vi "getAll.vi"(8 "error in (no error)":errorcluster, 11 "Instrument.Oxford1820 in":refnum<class "Instrument.OxfordVRM.lvclass">) -> (0 "error out":errorcluster, 2 "getAll":variant, 3 "Instrument.Oxford1820 out":refnum<class "Instrument.OxfordVRM.lvclass">)   [LabVIEW 2016, in "Instrument.OxfordVRM.lvclass"]
uses:
  Instrument.OxfordVRM.lvclass
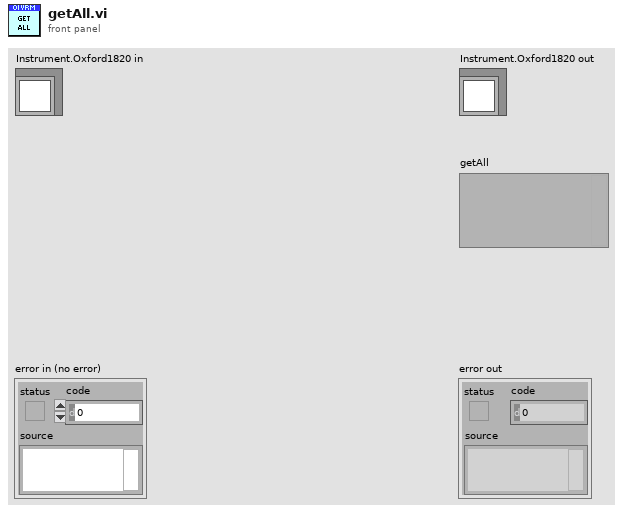
[diagram p1: front panel]
types:
  T1 = typedef "Instrument.OxfordVRM.lvclass/getAll.ctl" = cluster{"1820_IPS_Magnet_Field":dbl, "1820_IPS_PS_Field":dbl, "1820_IPS_Target_Field":dbl, "1820_IPS_Target_Field_Rate":dbl, "1820_IPS_Voltage":dbl, "1820_IPS_Current":dbl, "1820_IPS_Level_N2":dbl, "1820_IPS_Level_He":dbl, "1820_IPS_Magnet_Temperature":dbl, "1820_IPS_Magnet_Temperature_R":dbl, "1820_IPS_M1_Current":dbl, "1820_IPS_M1_Voltage":dbl, "1820_IPS_M2_Current":dbl, "1820_IPS_M2_Voltage":dbl, "1820_IPS_M3_Current":dbl, "1820_IPS_M3_Voltage":dbl, "1820_IPS_Status":string, "1820_IPS_Switch":string, "1820_ITC_Lambda_Temperature":dbl, "1820_ITC_Lambda_Temperature_R":dbl, "1820_ITC_Pressure":dbl, "1820_ITC_Needle_Valve":dbl}
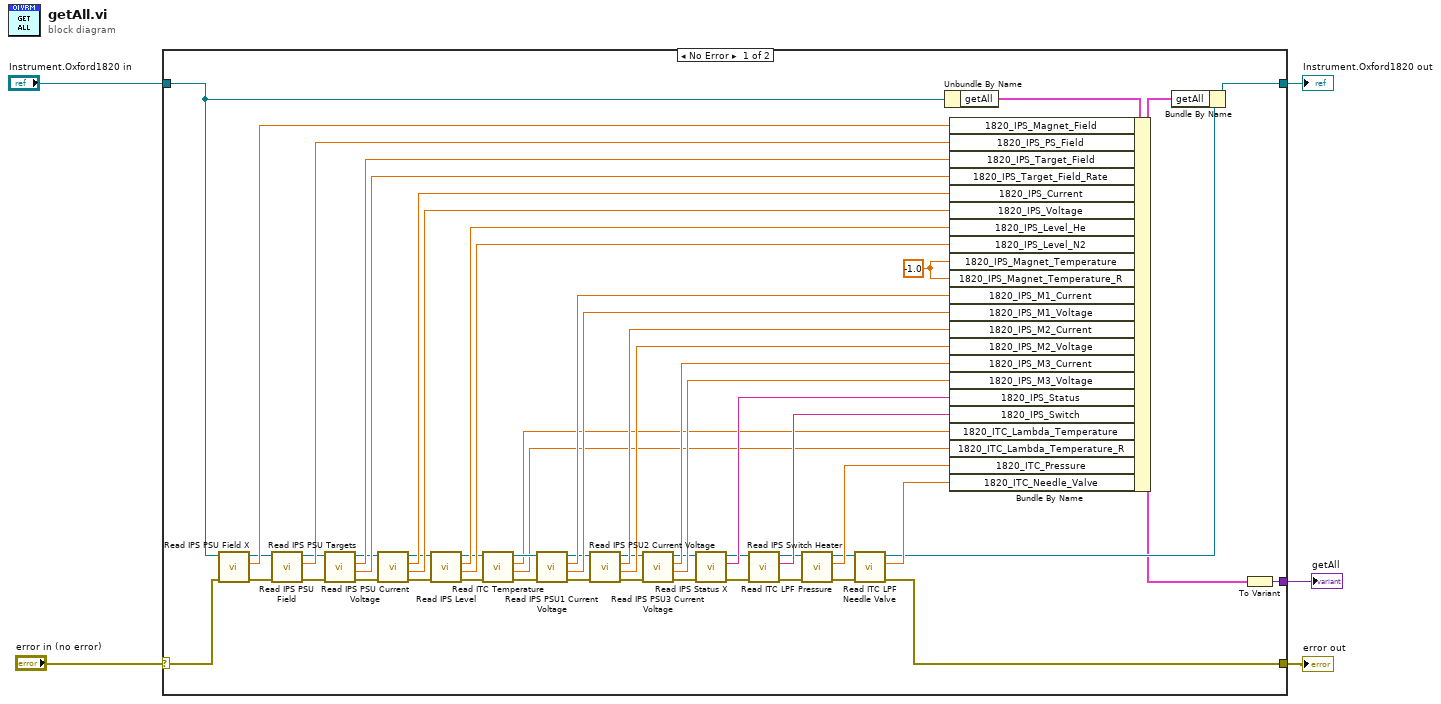
[diagram p0: block diagram]
diagram:
  n1 = case shown="No Error" "error in (no error)" {
    selector: "error in (no error)" -> [w40 w59]
    tunnel: "Instrument.Oxford1820 in" -> [w13 w60]
    tunnel: [w17 w60] -> w4
    tunnel: [w39 w59] -> w2
    tunnel: [w15 _] -> w1
    frame No Error {
      w8 = -1.0 ("getAll.1820_ITC_Lambda_Temperature")
      n2 = call "Read IPS PSU Field X.vi"("error in (no error)"=w40, "Instrument.OxfordVRM in"=w13) -> ("error out"=w37:errorcluster, "Magnet Field (T)"=w58:dbl, "Instrument.OxfordVRM out"=w38:refnum<class "Instrument.OxfordVRM.lvclass">)  [unwired: 7 in]
      n3 = call "Read IPS PSU Field.vi"("error in (no error)"=w37, "Instrument.OxfordVRM in"=w38) -> ("error out"=w35:errorcluster, "Power Supply Field (T)"=w57:dbl, "Instrument.OxfordVRM out"=w36:refnum<class "Instrument.OxfordVRM.lvclass">)  [unwired: 7 in]
      n4 = call "Read IPS PSU Targets.vi"("error in (no error)"=w35, "Instrument.OxfordVRM in"=w36) -> ("error out"=w33:errorcluster, "Target Field Rate (T/min)"=w55:dbl, "Target Field (T)"=w56:dbl, "Instrument.OxfordVRM out"=w34:refnum<class "Instrument.OxfordVRM.lvclass">)  [unwired: 6 in]
      n5 = call "Read IPS PSU Current Voltage.vi"("error in (no error)"=w33, "Instrument.OxfordVRM in"=w34) -> ("error out"=w31:errorcluster, "Voltage (V)"=w53:dbl, "Current (A)"=w54:dbl, "Instrument.OxfordVRM out"=w32:refnum<class "Instrument.OxfordVRM.lvclass">)  [unwired: 6 in]
      n6 = call "Read IPS Level.vi"("error in (no error)"=w31, "Instrument.Oxford1820 in"=w32) -> ("error out"=w11:errorcluster, "N2 Level (%)"=w51:dbl, "He Level (%)"=w52:dbl, "Instrument.Oxford1820 out"=w12:refnum<class "Instrument.OxfordVRM.lvclass">)  [unwired: 6 in]
      n7 = call "Read ITC Temperature.vi"("error in (no error)"=w11, "Instrument.Oxford1820 in"=w12) -> ("error out"=w10:errorcluster, "Resistance (Ohms)"=w6:dbl, "Temperature (K)"=w7:dbl, "Instrument.Oxford1820 out"=w9:refnum<class "Instrument.OxfordVRM.lvclass">)  [unwired: 6 in]
      n8 = call "Read IPS PSU1 Current Voltage.vi"("error in (no error)"=w10, "Instrument.OxfordVRM in"=w9) -> ("error out"=w29:errorcluster, "Voltage (V)"=w49:dbl, "Current (A)"=w50:dbl, "Instrument.OxfordVRM out"=w30:refnum<class "Instrument.OxfordVRM.lvclass">)  [unwired: 6 in]
      n9 = call "Read IPS PSU2 Current Voltage.vi"("error in (no error)"=w29, "Instrument.OxfordVRM in"=w30) -> ("error out"=w27:errorcluster, "Voltage (V)"=w47:dbl, "Current (A)"=w48:dbl, "Instrument.OxfordVRM out"=w28:refnum<class "Instrument.OxfordVRM.lvclass">)  [unwired: 6 in]
      n10 = call "Read IPS PSU3 Current Voltage.vi"("error in (no error)"=w27, "Instrument.OxfordVRM in"=w28) -> ("error out"=w25:errorcluster, "Voltage (V)"=w45:dbl, "Current (A)"=w46:dbl, "Instrument.OxfordVRM out"=w26:refnum<class "Instrument.OxfordVRM.lvclass">)  [unwired: 6 in]
      n11 = call "Read IPS Status X.vi"("error in (no error)"=w25, "Instrument.OxfordVRM in"=w26) -> ("error out"=w23:errorcluster, "Status"=w44:string, "Instrument.OxfordVRM out"=w24:refnum<class "Instrument.OxfordVRM.lvclass">)  [unwired: 7 in]
      n12 = call "Read IPS Switch Heater.vi"("error in (no error)"=w23, "Instrument.Oxford1820 in"=w24) -> ("error out"=w21:errorcluster, "Switch Heater Status"=w43:string, "Instrument.Oxford1820 out"=w22:refnum<class "Instrument.OxfordVRM.lvclass">)  [unwired: 6 in, 1 out]
      n13 = call "Read ITC LPF Pressure.vi"("error in (no error)"=w21, "Instrument.Oxford1820 in"=w22) -> ("error out"=w19:errorcluster, "LPF Pressure (mbar)"=w42:dbl, "Instrument.Oxford1820 out"=w20:refnum<class "Instrument.OxfordVRM.lvclass">)  [unwired: 7 in]
      n14 = call "Read ITC LPF Needle Valve.vi"("error in (no error)"=w19, "Instrument.Oxford1820 in"=w20) -> ("error out"=w39:errorcluster, "LPF Needle Valve (%)"=w41:dbl, "Instrument.Oxford1820 out"=w16:refnum<class "Instrument.OxfordVRM.lvclass">)  [unwired: 7 in]
      n15 = Unbundle By Name(w13) -> ("getAll"=w18:T1)
      n16 = Bundle By Name(cluster=w18, "1820_IPS_Magnet_Field"=w58, "1820_IPS_PS_Field"=w57, "1820_IPS_Target_Field"=w56, "1820_IPS_Target_Field_Rate"=w55, "1820_IPS_Current"=w54, "1820_IPS_Voltage"=w53, "1820_IPS_Level_He"=w52, "1820_IPS_Level_N2"=w51, "1820_IPS_Magnet_Temperature"=w8, "1820_IPS_Magnet_Temperature_R"=w8, "1820_IPS_M1_Current"=w50, "1820_IPS_M1_Voltage"=w49, "1820_IPS_M2_Current"=w48, "1820_IPS_M2_Voltage"=w47, "1820_IPS_M3_Current"=w46, "1820_IPS_M3_Voltage"=w45, "1820_IPS_Status"=w44, "1820_IPS_Switch"=w43, "1820_ITC_Lambda_Temperature"=w7, "1820_ITC_Lambda_Temperature_R"=w6, "1820_ITC_Pressure"=w42, "1820_ITC_Needle_Valve"=w41) -> (w14:T1)
      n17 = Bundle By Name(cluster=w16, "getAll"=w14) -> (w17:refnum<class "Instrument.OxfordVRM.lvclass">)
      n18 = To Variant(anything=w14) -> (Variant=w15:variant)
    }
    frame Error {
    }
  }
  "error out" <- w2
  "Instrument.Oxford1820 out" <- w4
  "getAll" <- w1
